vi "Set BC.vi"(6 "index":i32, 7 "target BC":refnum<class "NI_BC.lvclass">, 8 "error in (no error)":errorcluster, 9 "# of BC":i32, 10 "BC":variant, 11 "PDE in":refnum<class "NI_PDE.lvclass">) -> (0 "error out":errorcluster, 3 "PDE out":refnum<class "NI_PDE.lvclass">)   [LabVIEW 2020, in "NI_PDE.lvlib" / "NI_PDE.lvclass"]
uses:
  <vilib>/gmath/pde.llb/PDEClass/NI_PDE.lvclass
  <vilib>/gmath/pde.llb/BCClass/NI_BC.lvclass
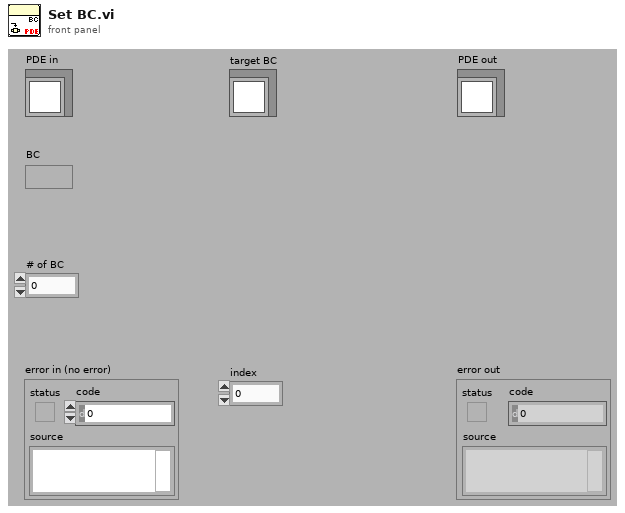
[diagram p1: front panel]
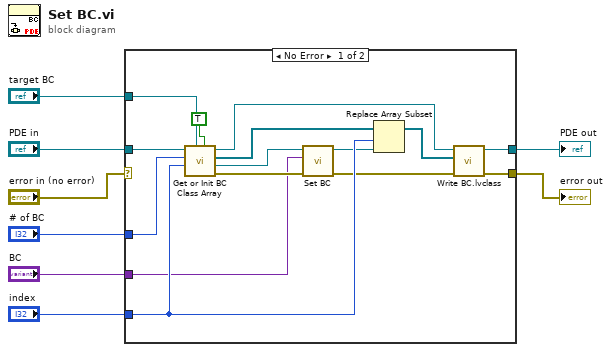
[diagram p0: block diagram]
diagram:
  n1 = case shown="No Error" "error in (no error)" {
    selector: "error in (no error)" -> [_ w25]
    tunnel: "PDE in" -> [w20 w24]
    tunnel: [w19 w24] -> w7
    tunnel: [w18 w25] -> w6
    tunnel: "BC" -> [w10 _]
    tunnel: "index" -> [w17 _]
    tunnel: "target BC" -> [w16 _]
    tunnel: "# of BC" -> [w11 _]
    frame No Error {
      n2 = call <vilib>:"Get or Init BC Class Array.vi"("type check? (T)"=TRUE, "target BC"=w16, "index"=w17, "# of BC"=w11, "PDE in"=w20) -> ("error out"=w12:errorcluster, "BC out"=w13:refnum<class "NI_BC.lvclass">, "BC Array"=w22:refnum<class "NI_BC.lvclass">[], "PDE out"=w21:refnum<class "NI_PDE.lvclass">)  [unwired: 1 in, 2 out]
      n3 = call-dynamic "Set BC.vi"("error in (no error)"=w12, "BC"=w10, "BC in"=w13) -> ("error out"=w14:errorcluster, "BC out"=w15:refnum<class "NI_BC.lvclass">)  [unwired: 7 out]
      n4 = Replace Array Subset(array=w22, new element=w15, index=w17) -> (w23:refnum<class "NI_BC.lvclass">[])
      n5 = call-dynamic "Write BC.lvclass.vi"("error in (no error)"=w14, "BC.lvclass"=w23, "PDE.lvclass in"=w21) -> ("error out"=w18:errorcluster, "PDE.lvclass out"=w19:refnum<class "NI_PDE.lvclass">)  [unwired: 7 out]
    }
    frame Error {
    }
  }
  "PDE out" <- w7
  "error out" <- w6
